vi "Check Parameters.vi"(8 "error in (no error)":errorcluster, 10 "Dynamic Model":bool, 11 "NI_Robotics_Serial Robot Arm in":refnum<class "NI_Robotics_Serial Robot Arm.lvclass">) -> (0 "error out":errorcluster, 3 "NI_Robotics_Serial Robot Arm out":refnum<class "NI_Robotics_Serial Robot Arm.lvclass">)   [LabVIEW 2017, in "NI_Robotics_Serial Robot Arm.lvclass"]
uses:
  <vilib>/robotics/Kinematics/Robot/NI_Robotics_Serial Robot Arm.lvclass
  <vilib>/robotics/Kinematics/Link/NI_Robotics_Link.lvclass
  <vilib>/robotics/Utilities/NI_Robotics Utilities.lvlib
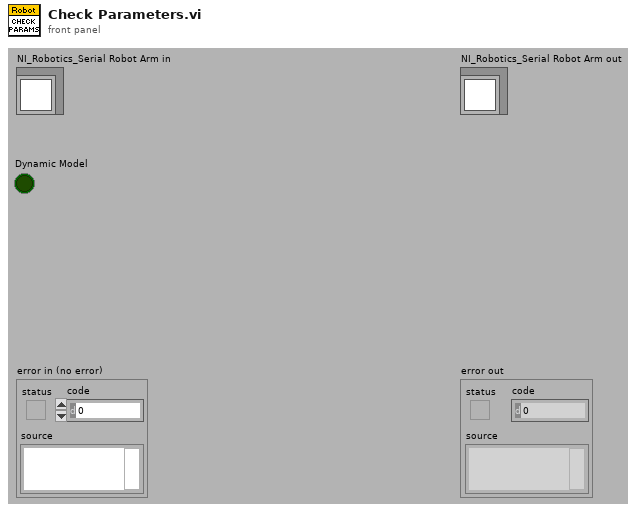
[diagram p1: front panel]
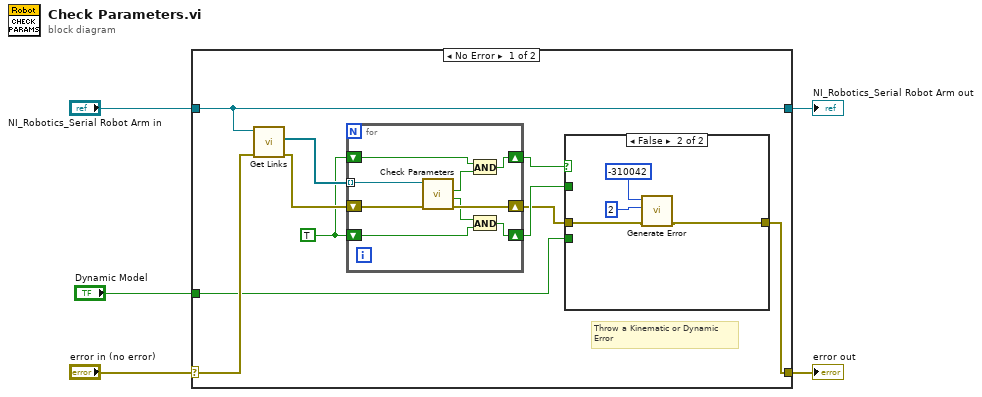
[diagram p0: block diagram]
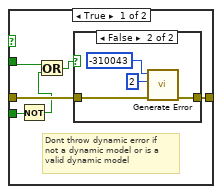
[diagram p2: hidden frame]
diagram:
  n1 = case shown="No Error" "error in (no error)" {
    selector: "error in (no error)" -> [w8 w41]
    tunnel: [w7 w41] -> w4
    tunnel: [w15 w40] -> w2
    tunnel: "NI_Robotics_Serial Robot Arm in" -> [w15 w40]
    tunnel: "Dynamic Model" -> [w6 _]
    frame No Error {
      w12 = TRUE
      # "Throw a Kinematic or Dynamic\nError"
      n2 = call <vilib>:"Get Links.vi"("error in (no error)"=w8, "serial arm in"=w15) -> ("error out"=w13:errorcluster, "links"=w14:refnum<class "NI_Robotics_Link.lvclass">[])  [unwired: 7 in, 1 out]
      n3 = for {
        tunnel: w14 -> [w39] mode=indexing
        shift-right: [w37] -> w9
        shift-left: w13 -> [w38]
        shift-right: [w31] -> w11
        shift-left: w12 -> [w34]
        shift-right: [w33] -> w10
        shift-left: w12 -> [w32]
        n4 = call-dynamic "Check Parameters.vi"("error in (no error)"=w38, "link in"=w39) -> ("error out"=w37:errorcluster, "dynamics valid"=w36:bool, "kinematics valid"=w35:bool)  [unwired: 6 in, 1 out]
        n5 = And(x=w34, y=w35) -> (x .and. y?=w31:bool)
        n6 = And(x=w36, y=w32) -> (x .and. y?=w33:bool)
      }
      n7 = case shown="False" w11 {
        tunnel: w9 -> [w21 w30]
        tunnel: [w20 w29] -> w7
        tunnel: w10 -> [w17 _]
        tunnel: w6 -> [w19 _]
        frame True {
          # "Dont throw dynamic error if\nnot a dynamic model or is a \nvalid dynamic model"
          n8 = Not(x=w19) -> (.not. x?=w16:bool)
          n9 = Or(x=w17, y=w16) -> (x .or. y?=w18:bool)
          n10 = case shown="False" w18 {
            tunnel: w21 -> [w22 w26]
            tunnel: [w22 w25] -> w20
            frame True {
            }
            frame False {
              n11 = call <vilib>:"Generate Error.vi"("error in (no error)"=w26, "chain levels to remove (1)"=2, "code"=-310043) -> ("error out"=w25:errorcluster)  [unwired: 8 in]
            }
          }
        }
        frame False {
          n12 = call <vilib>:"Generate Error.vi"("error in (no error)"=w30, "chain levels to remove (1)"=2, "code"=-310042) -> ("error out"=w29:errorcluster)  [unwired: 8 in]
        }
      }
    }
    frame Error {
    }
  }
  "error out" <- w4
  "NI_Robotics_Serial Robot Arm out" <- w2
